vi "Plot.vi"(8 "error in (no error)":errorcluster, 11 "Spectrum Recorder in":refnum<class "Spectrum Recorder too.lvclass">) -> (0 "error out":errorcluster, 3 "Spectrum Recorder out":refnum<class "Spectrum Recorder too.lvclass">)   [LabVIEW 2016, in "Spectrum Recorder too.lvclass"]
uses:
  Spectrum Recorder too.lvclass
  Spectrum Recorder too.lvclass/Spectrum Recorder too.ctl
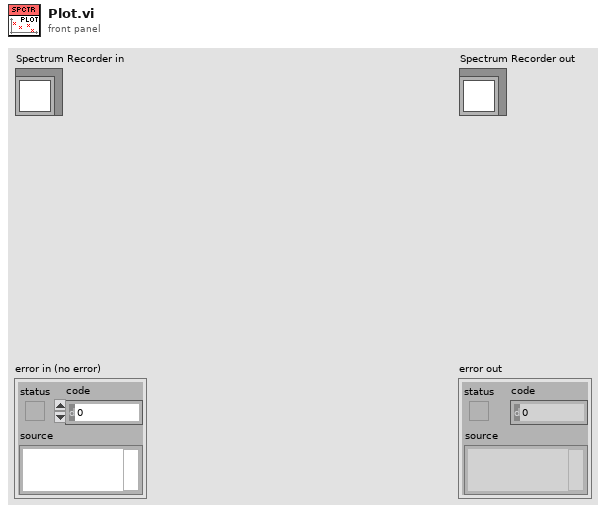
[diagram p1: front panel]
types:
  T1 = enum16{"open", "open or create", "create or replace", "create", "open (read-only)"}
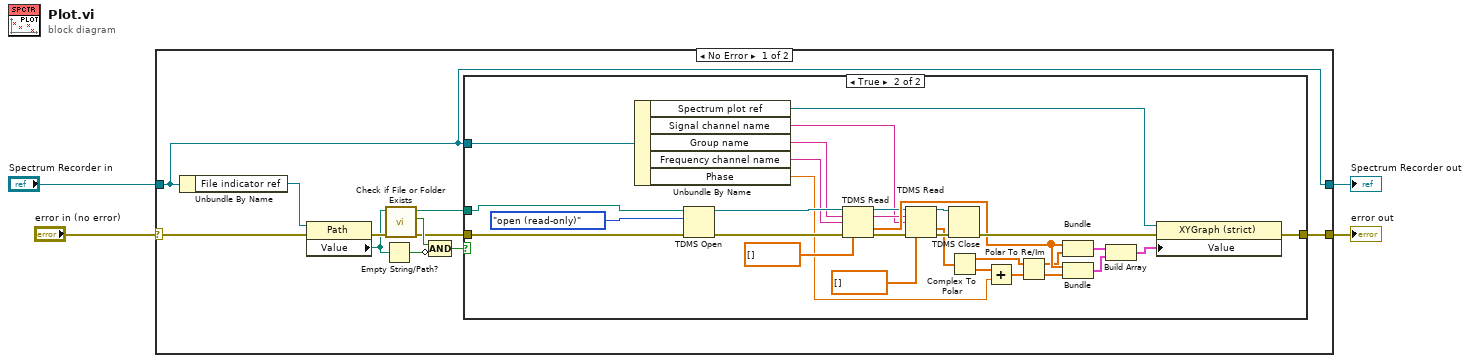
[diagram p0: block diagram]
diagram:
  n1 = case shown="No Error" "error in (no error)" {
    selector: "error in (no error)" -> [w6 w48]
    tunnel: [w5 w48] -> w3
    tunnel: [w7 w47] -> w1
    tunnel: "Spectrum Recorder in" -> [w7 w47]
    frame No Error {
      n2 = Unbundle By Name(w7) -> ("File indicator ref"=w15:refnum<vi>)
      n3 = property class="Path"(reference=w15, error in=w6) -> (error out=w14:errorcluster, "Value"=w13:path)  [unwired: 1 out]
      n4 = Empty String/Path?(string/path=w13) -> (empty?=w11:bool)
      n5 = call <vilib>:"Check if File or Folder Exists.vi"("error in (no error)"=w14, "path"=w13) -> ("error out"=w8:errorcluster, "file or folder exists?"=w12:bool, "dup path"=w9:path)  [unwired: 7 in]
      n6 = Compound Arithmetic op=AND(w12, invert w11) -> (w10:bool)
      n7 = case shown="True" w10 {
        tunnel: w9 -> [_ w44]
        tunnel: w8 -> [w16 w43]
        tunnel: w7 -> [_ w41]
        tunnel: [w16 w36] -> w5
        frame False {
        }
        frame True {
          n8 = Unbundle By Name(w41) -> ("Spectrum plot ref"=w35:refnum<vi>, "Signal channel name"=w25:string, "Group name"=w40:string, "Frequency channel name"=w39:string, "Phase"=w19:dbl)
          n9 = TDMS Open(8:w43, 10:T1."open (read-only)" ("operation (0:open)"), 11:w44) -> (0:w45:errorcluster, 3:w46:refnum<k34>)  [unwired: 4 in]
          n10 = TDMS Read(0:w46, 5:w40, 7:w39, 11:w45, 12:dbl[] []) -> (4:w30:refnum<k34>, 6:w26:string, 10:w31:dbl[], 15:w28:errorcluster)  [unwired: 3 in, 2 out]
          n11 = TDMS Read(0:w30, 5:w26, 7:w25, 11:w28, 12:cdb[] []) -> (4:w29:refnum<k34>, 10:w23:cdb[], 15:w27:errorcluster)  [unwired: 3 in, 3 out]
          n12 = TDMS Close(8:w27, 11:w29) -> (0:w37:errorcluster)  [unwired: 1 out]
          n13 = Complex To Polar(r * e^(i*theta)=w23) -> (r=w22:dbl[], theta=w21:dbl[])
          n14 = Add(x=w21, y=w19) -> (x+y=w20:dbl[])
          n15 = Polar To Re/Im(2:w20, 3:w22) -> (0:w17:dbl[], 1:w18:dbl[])
          n16 = Bundle(w31, w18) -> (w34:cluster{dbl[], dbl[]})  [unwired: 1 in]
          n17 = Bundle(w31, w17) -> (w33:cluster{dbl[], dbl[]})  [unwired: 1 in]
          n18 = Build Array(w34, w33) -> (w32:cluster{dbl[], dbl[]}[])
          n19 = property class="XYGraph (strict)"(reference=w35, error in=w37, "Value"=w32) -> (error out=w36:errorcluster)  [unwired: 1 out]
        }
      }
    }
    frame Error {
    }
  }
  "error out" <- w3
  "Spectrum Recorder out" <- w1
